vi "oa_SCL Draw Cursor and Label.vi"(5 "shaft center line settings":T5={"cartesian grid cosmetics"={"line color"=39168, "text color"=65280, "tick length(3)"=3, "crossing axes"=FALSE, "visible grid?"=TRUE}, "XY plot cosmetics"={"plot color"=16776960, "XY plot type"=enum."connected points", "baseline"=0.0}, "desired font(Application)"=enum."Application Font", "[user-specified font]"={"Font Name:"="", "Size"=0, "Strikeout?"=FALSE, "Italic?"=FALSE, "Underline?"=FALSE, "Outline?"=FALSE, "Shadow?"=FALSE, "Bold?"=FALSE}} {"XY plot cosmetics"."baseline" format="%0.2f"}, 6 "cursor attributes":T2={"layout color"=852223, "active color"=16740820, "precision"=2, "BG transparent? (T)"=FALSE, "radius"=2}, 8 "avoid overlap? (Y)":bool=TRUE, 9 "scale info":T1, 10 "Cursor List":T3(array[cluster]) {"Location"."Y" format="%.2f"; "Location"."X" format="%.2f"}, 11 "picture":picture) -> (3 "new picture":picture)   [LabVIEW 2017]
uses:
  <vilib>/picture/cartesn2.llb/XY Plot Type.ctl
  <vilib>/addons/Sound and Vibration/Order Analysis/Backward Compatibility/SubVIs/OAT Polar Cursor Attributes.ctl
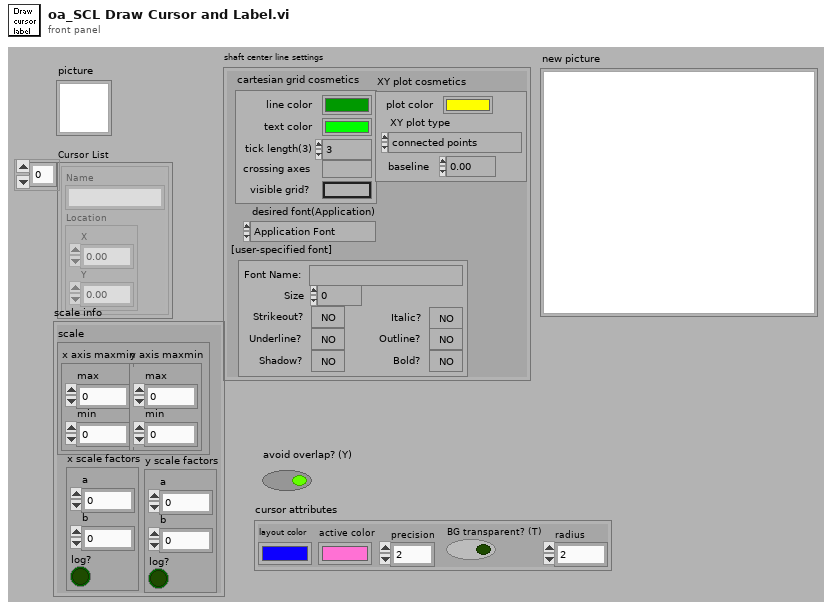
[diagram p1: front panel]
types:
  T1 = cluster{"scale":cluster{"x axis maxmin":cluster{"max":dbl, "min":dbl}, "y axis maxmin":cluster{"max":dbl, "min":dbl}}, "x scale factors":cluster{"a":dbl, "b":dbl, "log?":bool}, "y scale factors":cluster{"a":dbl, "b":dbl, "log?":bool}}
  T2 = typedef "OAT Polar Cursor Attributes.ctl" = cluster{"layout color":u32, "active color":u32, "precision":i16, "BG transparent? (T)":bool, "radius":i16}
  T3 = cluster{"Name":string, "Location":cluster{"X":dbl, "Y":dbl}}[]
  T4 = typedef "XY Plot Type.ctl" = enum16{"points", "squares", "circles", "connected points", "connected squares", "connected circles", "comb plot", "sized scatter plot", "sized-colored scatter plot", "min-max lines"}
  T5 = cluster{"cartesian grid cosmetics":cluster{"line color":u32, "text color":u32, "tick length(3)":i16, "crossing axes":bool, "visible grid?":bool}, "XY plot cosmetics":cluster{"plot color":u32, "XY plot type":T4, "baseline":dbl}, "desired font(Application)":enum16{"User-specified Font", "Application Font", "System Font", "Dialog Font"}, "[user-specified font]":cluster{"Font Name:":string, "Size":i16, "Strikeout?":bool, "Italic?":bool, "Underline?":bool, "Outline?":bool, "Shadow?":bool, "Bold?":bool}}
  T6 = cluster{"left":i16, "top":i16, "right":i16, "bottom":i16}[]
  T7 = enum16{"User-specified Font", "Application Font", "System Font", "Dialog Font"}
  T8 = cluster{"Font Name:":string, "Size":i16, "Strikeout?":bool, "Italic?":bool, "Underline?":bool, "Outline?":bool, "Shadow?":bool, "Bold?":bool}
  T9 = cluster{"left":i16, "top":i16, "right":i16, "bottom":i16}
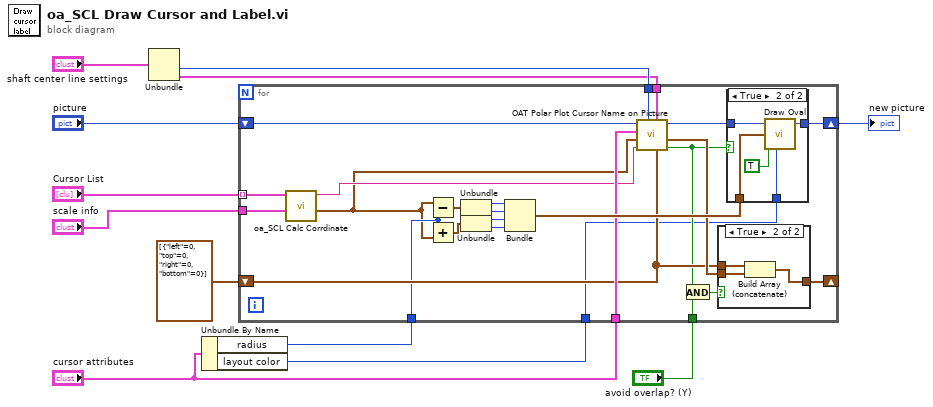
[diagram p0: block diagram]
diagram:
  n1 = Unbundle("shaft center line settings") -> ("desired font(Application)"=w3:T7, "[user-specified font]"=w1:T8)  [unwired: 2 out]
  n2 = Unbundle By Name("cursor attributes") -> ("radius"=w5:i16, "layout color"=w11:u32)
  n3 = for {
    tunnel: "Cursor List" -> [w16] mode=indexing
    shift-right: [w28] -> w10
    shift-left: "picture" -> [w27]
    tunnel: w11 -> [w26]
    tunnel: w5 -> [w25]
    tunnel: w3 -> [w15]
    tunnel: "cursor attributes" -> [w36]
    shift-right: [w32] -> _
    shift-left: T6 [{"left"=0, "top"=0, "right"=0, "bottom"=0}] -> [w31]
    tunnel: "avoid overlap? (Y)" -> [w34]
    tunnel: "scale info" -> [w13]
    tunnel: w1 -> [w14]
    n4 = call <vilib>:"oa_SCL Calc Corrdinate.vi"("scale info"=w13, "cursor list"=w16) -> ("position"=w17:cluster{"x":i16, "y":i16}, "Name"=w18:string)  [unwired: 8 in]
    n5 = Subtract(x=w17, y=w25) -> (x-y=w23:cluster{"x":i16, "y":i16})
    n6 = Add(x=w25, y=w17) -> (x+y=w24:cluster{"x":i16, "y":i16})
    n7 = Unbundle(w23) -> ("x"=w22:i16, "y"=w21:i16)
    n8 = Unbundle(w24) -> ("x"=w20:i16, "y"=w19:i16)
    n9 = Bundle("x"=w22, "y"=w21, "x"=w20, "y"=w19) -> (w37:cluster{"x":i16, "y":i16, "x":i16, "y":i16})  [unwired: 1 in]
    n10 = call <vilib>:"OAT Polar Plot Cursor Name on Picture.vi"("avoid rect"=w31, "[user-specified font]"=w14, "desired font(Application)"=w15, "name"=w18, "cursor position"=w17, "cursor attributes"=w36, "picture"=w27) -> ("text plotted"=w30:bool, "text rect"=w33:T9, "new picture"=w29:picture)  [unwired: 2 in]
    n11 = And(x=w30, y=w34) -> (x .and. y?=w35:bool)
    n12 = case shown="True" w35 {
      tunnel: w33 -> [_ w47]
      tunnel: [w44 w46] -> w32
      tunnel: w31 -> [w44 w45]
      frame False {
      }
      frame True {
        n13 = Build Array (concatenate)(w45, w47) -> (w46:T6)
      }
    }
    n14 = case shown="True" w30 {
      tunnel: w29 -> [w38 w43]
      tunnel: [w38 w42] -> w28
      tunnel: w37 -> [_ w41]
      tunnel: w26 -> [_ w40]
      frame False {
      }
      frame True {
        n15 = call <vilib>:"Draw Oval.vi"("picture"=w43, "rect"=w41, "fill?(F)"=TRUE, "color(black)"=w40) -> ("new picture"=w42:picture)  [unwired: 5 in]
      }
    }
  }
  "new picture" <- w10
